vi "RAMP_move_to_new_Z_position.vi"(4 "error in":errorcluster, 6 "Z":dbl, 7 "queue piezo":refnum<queue>) -> (0 "error out":errorcluster, 3 "z":dbl)   [LabVIEW 2015]
uses:
  CONTROLS/Q_MCL_piezo_element.ctl
  GLOBAL/Global_MCL_piezo.vi
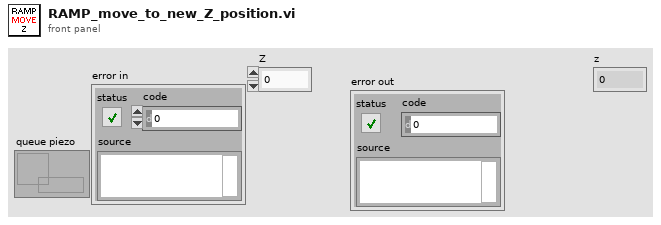
[diagram p1: front panel]
types:
  T1 = typedef "Q_MCL_piezo_element.ctl" = cluster{"variant":variant, "Instruction":enum16{"Piezo_idle", "Piezo_initialize", "Piezo_error", "Piezo_security_stop", "Piezo_read_z", "Piezo_move_z", "Piezo_keyboard_move", "Piezo_close_autofocus_calibration_ramp", "Piezo_change_init_state", "Piezo_init_autofocus", "Piezo_init_autofocus_merFISH_TL", "Piezo_autofocus", "Piezo_autofocus_merFISH_TL", "Piezo_stop_autofocus", "Piezo_stop_autofocus_merFISH_TL", "Piezo_autofocus_lost", "Piezo_resume_autofocus_merFISH_TL", "Piezo_check_z_position_merFISH_TL", "Piezo_init_ramp", "Piezo_move_z_ramp", "Piezo_close_ramp", "Piezo_close_merFISH", "Piezo_stop"}}
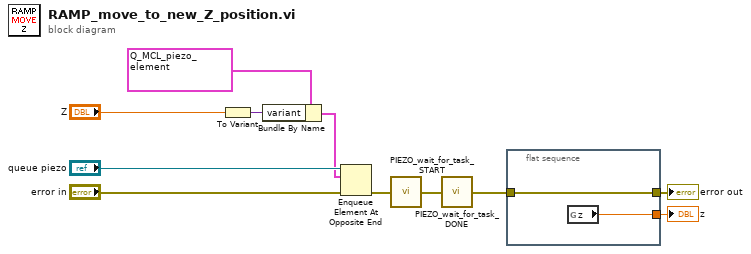
[diagram p0: block diagram]
diagram:
  n1 = To Variant(anything="Z") -> (Variant=w6:variant)
  n2 = Bundle By Name(cluster=T1 {"variant"=variant, "Instruction"=enum."Piezo_move_z"} ("element"), "variant"=w6) -> (w4:T1)
  n3 = Enqueue Element At Opposite End(queue="queue piezo", element=w4, error in (no error)="error in") -> (error out=w9:errorcluster)  [unwired: 1 in, 2 out]
  n4 = call "PIEZO_wait_for_task_START.vi"("error in"=w9) -> ("error out"=w8:errorcluster)
  n5 = call "PIEZO_wait_for_task_DONE.vi"("error in"=w8) -> ("error out"=w3:errorcluster)
  n6 = flat-sequence {
    tunnel: w3 -> [w13]
    tunnel: [w13] -> w2
    tunnel: [w12] -> w1
    frame #0 {
      n7 = global read "Global_MCL_piezo.vi" "z"() -> (w12:dbl)
    }
  }
  "error out" <- w2
  "z" <- w1
